vi "Insert Panel.vi"(8 "error in (no error)":errorcluster, 9 "Position (End)":i32=-1, 10 "Panel/Type":refnum<class "ArrayPanel.lvclass">, 11 "PanelArray in":refnum<class "ArrayManager.lvclass">) -> (0 "error out":errorcluster, 2 "Panel":refnum<class "ArrayPanel.lvclass">, 3 "PanelArray out":refnum<class "ArrayManager.lvclass">)   [LabVIEW 2020, in "OOPanel.lvlib" / "ArrayManager.lvclass"]
uses:
  <vilib>/IlluminatedG/IG OOPanel/OOPanel/ArrayManager/ArrayManager.lvclass
  <vilib>/IlluminatedG/IG OOPanel/OOPanel/ArrayPanel/ArrayPanel.lvclass
  C:/Program Files (x86)/National Instruments/LabVIEW 2020/vi.lib/IlluminatedG/IG OOPanel/OOPanel/Panel/Panel.lvclass
  <vilib>/IlluminatedG/IG OOPanel/OOPanel/Panel/Panel.lvclass/Panel.ctl
  <vilib>/IlluminatedG/IG OOPanel/OOPanel/ArrayManager/ArrayManager.lvclass/ArrayManager.ctl
  <vilib>/IlluminatedG/IG OOPanel/OOPanel/ArrayPanel/ArrayPanel.lvclass/ArrayPanel.ctl
  <vilib>/Utility/error.llb/Error Cluster From Error Code.vi
  <vilib>/ErrorRing/Error Ring.xnode
  <vilib>/IlluminatedG/IG OOPanel/OOPanel/Panel/Panel.lvclass
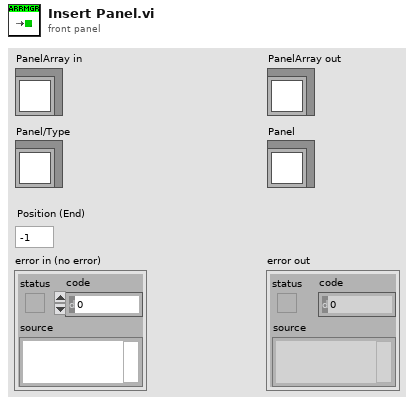
[diagram p1: front panel]
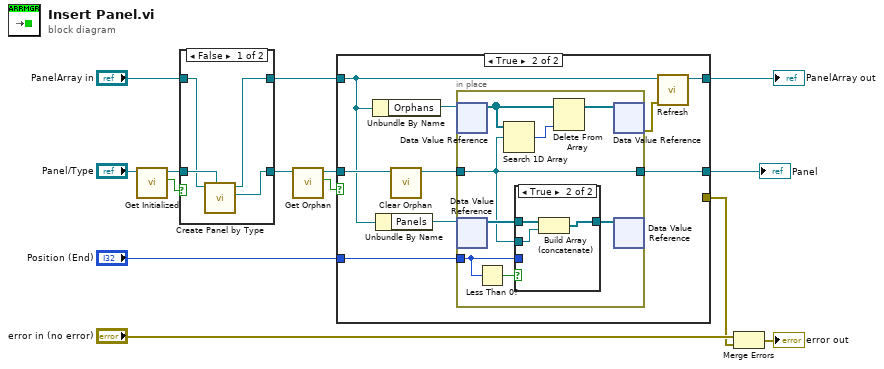
[diagram p0: block diagram]
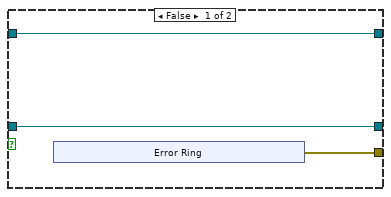
[diagram p3: hidden frame]
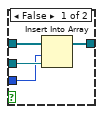
[diagram p4: hidden frame]
diagram:
  n1 = call <vilib>:"Get Initialized.vi"("Panel in"="Panel/Type") -> ("Initialized"=w6:bool, "Panel out"=w5:refnum<class "ArrayPanel.lvclass">)  [unwired: 8 in, 1 out]
  n2 = case shown="False" w6 {
    tunnel: w5 -> [w18 w20]
    tunnel: [w15 w20] -> w4
    tunnel: "PanelArray in" -> [w17 w19]
    tunnel: [w16 w19] -> w2
    frame False {
      n3 = call <vilib>:"Create Panel by Type.vi"("Panel Type"=w18, "PanelArray in"=w17) -> ("Panel"=w15:refnum<class "ArrayPanel.lvclass">, "PanelArray out"=w16:refnum<class "ArrayManager.lvclass">)  [unwired: 7 in, 1 out]
    }
    frame True {
    }
  }
  n4 = call <vilib>:"Get Orphan.vi"("ArrayPanel in"=w4) -> ("Orphan"=w13:bool, "ArrayPanel out"=w12:refnum<class "ArrayPanel.lvclass">)  [unwired: 8 in, 1 out]
  n5 = case shown="True" w13 {
    tunnel: w2 -> [w22 w30]
    tunnel: w12 -> [w21 w35]
    tunnel: [w23 _] -> w9
    tunnel: "Position (End)" -> [_ w33]
    tunnel: [w22 w31] -> w8
    tunnel: [w21 w28] -> w1
    frame False {
      n6 = xnode "Error Ring"() -> ("error out"=w23:errorcluster)
    }
    frame True {
      n7 = Unbundle By Name(w30) -> ("Orphans"=w36:refnum<data-value>)
      n8 = Unbundle By Name(w30) -> ("Panels"=w34:refnum<data-value>)
      n9 = call <vilib>:"Clear Orphan.vi"("ArrayPanel in"=w35) -> ("ArrayPanel out"=w29:refnum<class "ArrayPanel.lvclass">)  [unwired: 9 in, 1 out]
      n10 = in-place {
        in-place-border: w29 -> [w37]
        in-place-border: w33 -> [w39]
        in-place-border: [w37] -> w28
        n11 = in-place-dvr #1(w36) -> (w44:refnum<class "ArrayPanel.lvclass">[])  [unwired: 1 out]
        n12 = in-place-dvr #2(w34) -> (w41:refnum<class "ArrayPanel.lvclass">[])  [unwired: 1 out]
        n13 = Less Than 0?(x=w39) -> (x < 0?=w38:bool)
        n14 = Search 1D Array(1D array=w44, element=w37) -> (index of element=w42:i32)  [unwired: 1 in]
        n15 = case shown="True" w38 {
          tunnel: w39 -> [w46 _]
          tunnel: w41 -> [w48 w51]
          tunnel: w37 -> [w47 w50]
          tunnel: [w45 w49] -> w40
          frame False {
            n16 = Insert Into Array(array=w48, index=w46, new element=w47) -> (w45:refnum<class "ArrayPanel.lvclass">[])
          }
          frame True {
            n17 = Build Array (concatenate)(w51, w50) -> (w49:refnum<class "ArrayPanel.lvclass">[])
          }
        }
        n18 = Delete From Array(array=w44, index=w42) -> (array with subset deleted=w43:refnum<class "ArrayPanel.lvclass">[])  [unwired: 1 in, 1 out]
        n19 = in-place-dvr #1(w43) -> (w32:errorcluster)  [unwired: 1 out]
        n20 = in-place-dvr #2(w40) -> ()  [unwired: 2 out]
      }
      n21 = call <vilib>:"Refresh.vi"("error in (no error)"=w32, "ArrayManager in"=w30) -> ("ArrayManager out"=w31:refnum<class "ArrayManager.lvclass">)  [unwired: 8 in, 1 out]
    }
  }
  "PanelArray out" <- w8
  "Panel" <- w1
  n22 = Merge Errors("error in (no error)", w9) -> (→"error out":errorcluster)
